vi "PS4 Controller - Event Read.vi"() -> ()   [LabVIEW 2020, in "LMH-PS4.lvlib"]
doc: "This example demonstrates how to read from a Play Station 4 controller using events."
uses:
  LMH-PS4.lvlib
  Private/Type Defs/Axis.ctl
  Private/Type Defs/Indicators/DPad Enum.ctl
  Public/Open First Controller.vi
panel:
  out "All Axis":T1
  out "Event Log":string[](array[string])
  in  "Stop Button":bool
  # "Controller Data"
  # "PS4 Controller  - Event Based Read\n\nThis example demonstrates how to read all buttons and axis data from an PS4 controller using events.\n\nInstructions\n1. Connect the PS4 controller to the PC and make sure the drivers are installed.\n2. Click the Run Arrow.\n3. Notice the controller data on the front panel update to match the actual controller state."
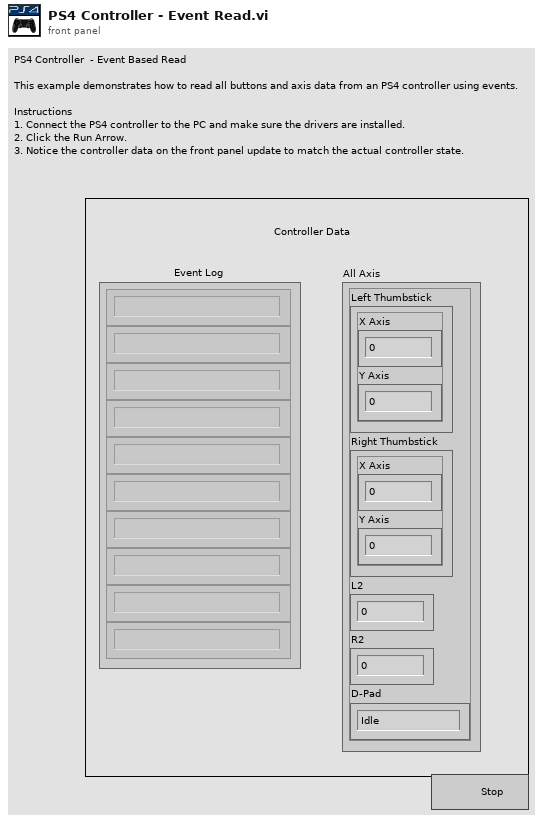
[diagram p1: front panel]
types:
  T1 = typedef "LMH-PS4.lvlib/Axis.ctl" = cluster{"Left Thumbstick":cluster{"X Axis":i32, "Y Axis":i32}, "Right Thumbstick":cluster{"X Axis":i32, "Y Axis":i32}, "L2":i32, "R2":i32, "D-Pad":T2}
  T2 = typedef "LMH-PS4.lvlib/DPad Enum.ctl" = enum16{"Idle", "Up", "Up / Right", "Right", "Down / Right", "Down", "Down / Left", "Left", "Up / Left"}
  T3 = typedef "LMH-PS4.lvlib/PS4 Controller Ref.ctl" = cluster{"Controller Ref":refnum<k1>, "PS4 Events Ref":refnum<event-registration>, "Worker Ref":refnum<vi>}
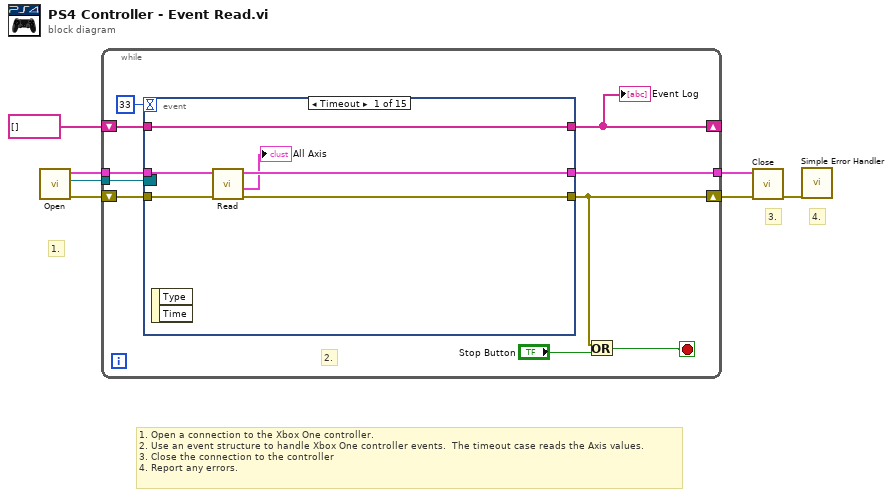
[diagram p0: block diagram]
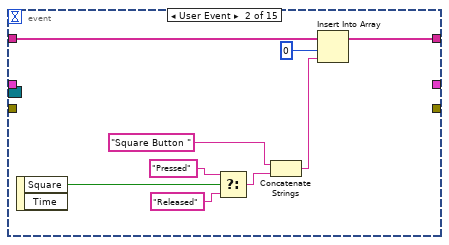
[diagram p2: hidden frame]
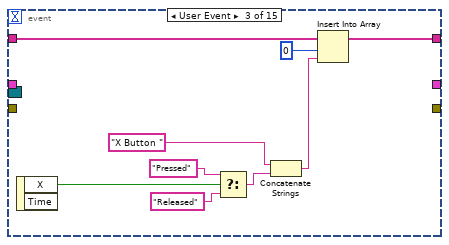
[diagram p3: hidden frame]
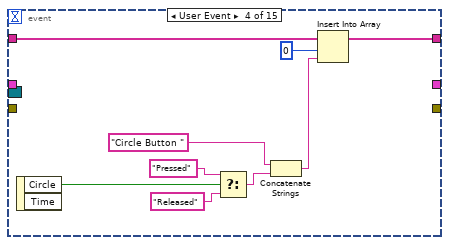
[diagram p4: hidden frame]
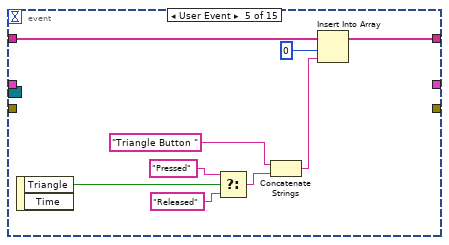
[diagram p5: hidden frame]
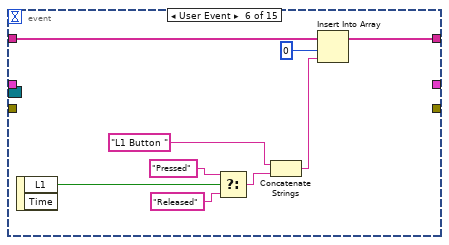
[diagram p6: hidden frame]
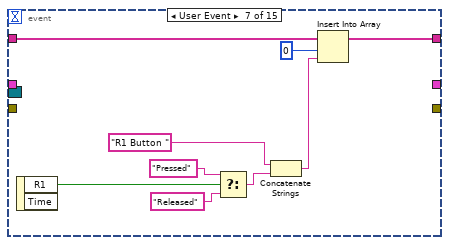
[diagram p7: hidden frame]
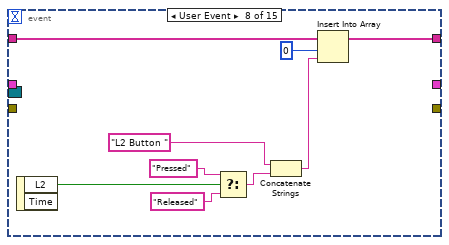
[diagram p8: hidden frame]
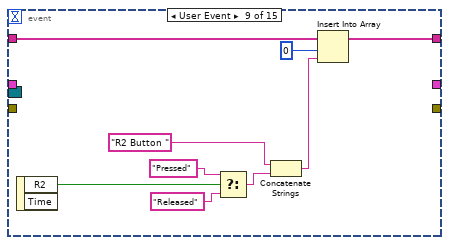
[diagram p9: hidden frame]
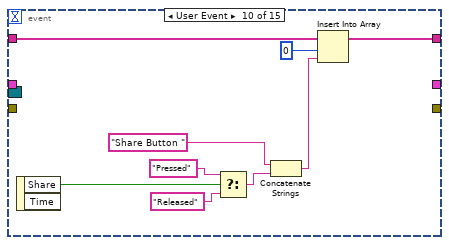
[diagram p10: hidden frame]
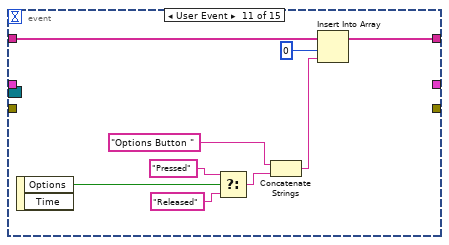
[diagram p11: hidden frame]
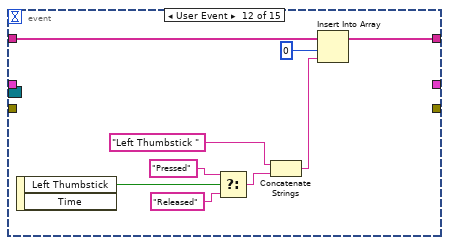
[diagram p12: hidden frame]
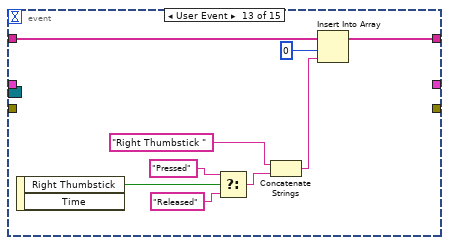
[diagram p13: hidden frame]
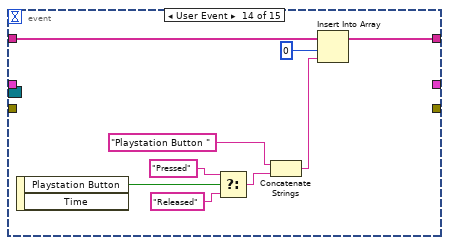
[diagram p14: hidden frame]
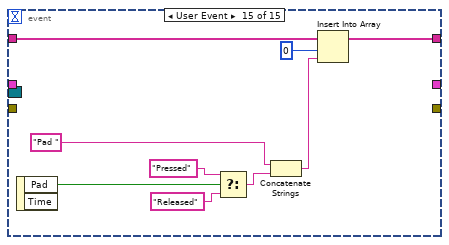
[diagram p15: hidden frame]
diagram:
  # "4."
  # "3."
  # "1."
  # "1. Open a connection to the Xbox One controller.\n2. Use an event structure to handle Xbox One controller events.  The timeout case reads the Axis values.\n3. Close the connection to the controller\n4. Report any errors."
  n1 = call-poly "Open.vi"() -> ("Error Out"=w5:errorcluster, "Event Registration Refnum"=w3:refnum<event-registration>, "PS4 Controller Ref"=w4:T3)  [unwired: 9 in]
  n2 = while {
    shift-right: [w13] -> w7
    shift-left: w5 -> [w16]
    tunnel: w4 -> [w17]
    tunnel: [w12] -> w6
    tunnel: w3 -> [w10]
    shift-right: [w8] -> _
    shift-left: string[] [] ("Event Log") -> [w9]
    stop <- w15 stop-if-true
    # "2."
    n3 = event shown="[0] Timeout" {
      selector: w10 -> [_ _ _ _ _ _ _ _ _ _ _ _ _ _ _]
      dyn-events: _ -> [_ _ _ _ _ _ _ _ _ _ _ _ _ _ _]
      timeout: 33 -> [_ _ _ _ _ _ _ _ _ _ _ _ _ _ _]
      tunnel: w17 -> [w22 _ _ _ _ _ _ _ _ _ _ _ _ _ _]
      tunnel: w16 -> [w21 _ _ _ _ _ _ _ _ _ _ _ _ _ _]
      tunnel: [w20 _ _ _ _ _ _ _ _ _ _ _ _ _ _] -> w13
      tunnel: [w19 _ _ _ _ _ _ _ _ _ _ _ _ _ _] -> w12
      tunnel: w9 -> [w23 w32 w41 w50 w59 w68 w77 w86 w95 w104 w113 w122 w131 w140 w149]
      tunnel: [w23 w24 w33 w42 w51 w60 w69 w78 w87 w96 w105 w114 w123 w132 w141] -> w8
      event Timeout {
        n4 = event-data() -> ()  [unwired: 1 in, 2 out]
        n5 = call "Read.vi"("Error In"=w21, "PS4 Controller Ref"=w22) -> ("Error Out"=w20:errorcluster, "All Axis"=→"All Axis":T1, "PS4 Controller Ref"=w19:T3)  [unwired: 6 in, 1 out]
      }
      event User Event {
        n6 = event-data() -> ("Square"=w31:bool)  [unwired: 1 in, 1 out]
        n7 = Select(t="Pressed", s=w31, f="Released") -> (s? t:f=w29:string)
        n8 = Concatenate Strings("Square Button ", w29) -> (w26:string)
        n9 = Insert Into Array(array=w32, index=0, new element=w26) -> (w24:string[])
      }
      event User Event {
        n10 = event-data() -> ("X"=w40:bool)  [unwired: 1 in, 1 out]
        n11 = Select(t="Pressed", s=w40, f="Released") -> (s? t:f=w38:string)
        n12 = Concatenate Strings("X Button ", w38) -> (w35:string)
        n13 = Insert Into Array(array=w41, index=0, new element=w35) -> (w33:string[])
      }
      event User Event {
        n14 = event-data() -> ("Circle"=w49:bool)  [unwired: 1 in, 1 out]
        n15 = Select(t="Pressed", s=w49, f="Released") -> (s? t:f=w47:string)
        n16 = Concatenate Strings("Circle Button ", w47) -> (w44:string)
        n17 = Insert Into Array(array=w50, index=0, new element=w44) -> (w42:string[])
      }
      event User Event {
        n18 = event-data() -> ("Triangle"=w58:bool)  [unwired: 1 in, 1 out]
        n19 = Select(t="Pressed", s=w58, f="Released") -> (s? t:f=w56:string)
        n20 = Concatenate Strings("Triangle Button ", w56) -> (w53:string)
        n21 = Insert Into Array(array=w59, index=0, new element=w53) -> (w51:string[])
      }
      event User Event {
        n22 = event-data() -> ("L1"=w67:bool)  [unwired: 1 in, 1 out]
        n23 = Select(t="Pressed", s=w67, f="Released") -> (s? t:f=w65:string)
        n24 = Concatenate Strings("L1 Button ", w65) -> (w62:string)
        n25 = Insert Into Array(array=w68, index=0, new element=w62) -> (w60:string[])
      }
      event User Event {
        n26 = event-data() -> ("R1"=w76:bool)  [unwired: 1 in, 1 out]
        n27 = Select(t="Pressed", s=w76, f="Released") -> (s? t:f=w74:string)
        n28 = Concatenate Strings("R1 Button ", w74) -> (w71:string)
        n29 = Insert Into Array(array=w77, index=0, new element=w71) -> (w69:string[])
      }
      event User Event {
        n30 = event-data() -> ("L2"=w85:bool)  [unwired: 1 in, 1 out]
        n31 = Select(t="Pressed", s=w85, f="Released") -> (s? t:f=w83:string)
        n32 = Concatenate Strings("L2 Button ", w83) -> (w80:string)
        n33 = Insert Into Array(array=w86, index=0, new element=w80) -> (w78:string[])
      }
      event User Event {
        n34 = event-data() -> ("R2"=w94:bool)  [unwired: 1 in, 1 out]
        n35 = Select(t="Pressed", s=w94, f="Released") -> (s? t:f=w92:string)
        n36 = Concatenate Strings("R2 Button ", w92) -> (w89:string)
        n37 = Insert Into Array(array=w95, index=0, new element=w89) -> (w87:string[])
      }
      event User Event {
        n38 = event-data() -> ("Share"=w103:bool)  [unwired: 1 in, 1 out]
        n39 = Select(t="Pressed", s=w103, f="Released") -> (s? t:f=w101:string)
        n40 = Concatenate Strings("Share Button ", w101) -> (w98:string)
        n41 = Insert Into Array(array=w104, index=0, new element=w98) -> (w96:string[])
      }
      event User Event {
        n42 = event-data() -> ("Options"=w112:bool)  [unwired: 1 in, 1 out]
        n43 = Select(t="Pressed", s=w112, f="Released") -> (s? t:f=w110:string)
        n44 = Concatenate Strings("Options Button ", w110) -> (w107:string)
        n45 = Insert Into Array(array=w113, index=0, new element=w107) -> (w105:string[])
      }
      event User Event {
        n46 = event-data() -> ("Left Thumbstick"=w121:bool)  [unwired: 1 in, 1 out]
        n47 = Select(t="Pressed", s=w121, f="Released") -> (s? t:f=w119:string)
        n48 = Concatenate Strings("Left Thumbstick ", w119) -> (w116:string)
        n49 = Insert Into Array(array=w122, index=0, new element=w116) -> (w114:string[])
      }
      event User Event {
        n50 = event-data() -> ("Right Thumbstick"=w130:bool)  [unwired: 1 in, 1 out]
        n51 = Select(t="Pressed", s=w130, f="Released") -> (s? t:f=w128:string)
        n52 = Concatenate Strings("Right Thumbstick ", w128) -> (w125:string)
        n53 = Insert Into Array(array=w131, index=0, new element=w125) -> (w123:string[])
      }
      event User Event {
        n54 = event-data() -> ("Playstation Button"=w139:bool)  [unwired: 1 in, 1 out]
        n55 = Select(t="Pressed", s=w139, f="Released") -> (s? t:f=w137:string)
        n56 = Concatenate Strings("Playstation Button ", w137) -> (w134:string)
        n57 = Insert Into Array(array=w140, index=0, new element=w134) -> (w132:string[])
      }
      event User Event {
        n58 = event-data() -> ("Pad"=w148:bool)  [unwired: 1 in, 1 out]
        n59 = Select(t="Pressed", s=w148, f="Released") -> (s? t:f=w146:string)
        n60 = Concatenate Strings("Pad ", w146) -> (w143:string)
        n61 = Insert Into Array(array=w149, index=0, new element=w143) -> (w141:string[])
      }
    }
    "Event Log" <- w8
    n62 = Or(x=w13, y="Stop Button") -> (x .or. y?=w15:bool)
  }
  n63 = call "Close.vi"("Error In"=w7, "PS4 Controller Ref"=w6) -> ("Error Out"=w1:errorcluster)  [unwired: 9 in]
  n64 = call <vilib>:"Simple Error Handler.vi"("error in (no error)"=w1) -> ()  [unwired: 4 in, 5 out]
